vi "DMControl_ae.vi"(1 "Enum":enum16{"WRITE", "READ"}(ring), 7 "Control":T1 {"Modes"."Amplititude" step=0.05}) -> (8 "Abberation Cluster Out":T1 {"Modes"."Amplititude" step=0.05})   [LabVIEW 2014]
uses:
  DMControl_STED.ctl
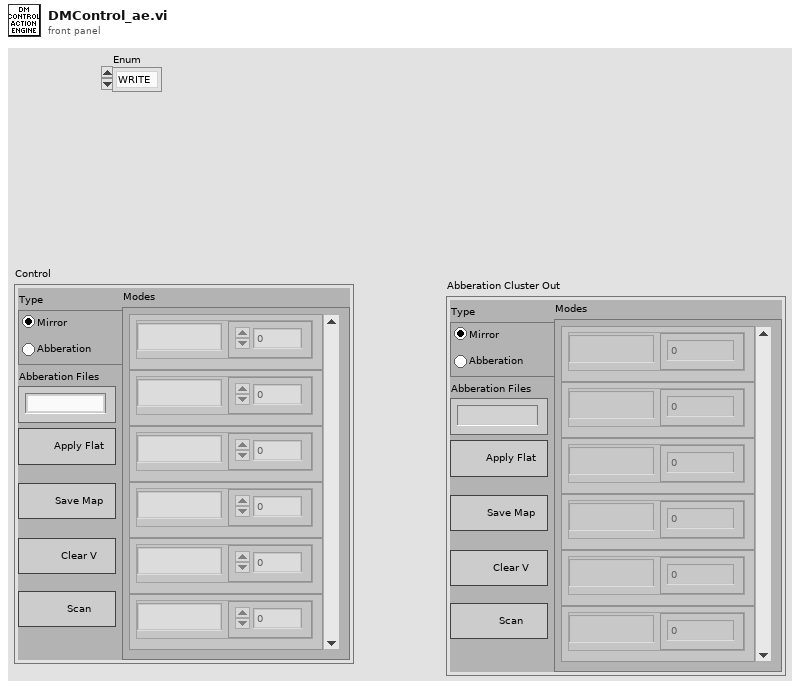
[diagram p1: front panel]
types:
  T1 = typedef "DMControl_STED.ctl" = cluster{"Type":enum32{"Mirror", "Abberation"}, "Modes":cluster{"Mode":string, "Amplititude":dbl}[], "Apply Flat":bool, "Save Map":bool, "Clear Voltage":bool, "Abberation Files":u16, "Scan ":bool}
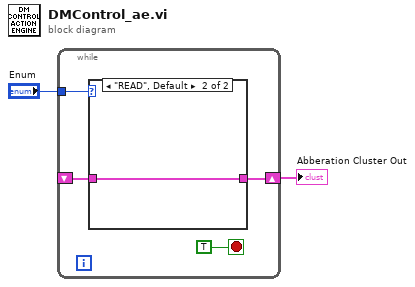
[diagram p0: block diagram]
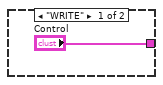
[diagram p2: hidden frame]
diagram:
  n1 = while {
    tunnel: "Enum" -> [w5]
    shift-right: [w4] -> w1
    shift-left: _ -> [w3]
    stop <- TRUE stop-if-true
    n2 = case shown="\"READ\", Default" w5 {
      tunnel: ["Control" w8] -> w4
      tunnel: w3 -> [_ w8]
      frame "WRITE" {
      }
      frame "READ", Default {
      }
    }
  }
  "Abberation Cluster Out" <- w1
